vi "loadSTL.vi"(10 "STLname":string, 11 "Job Directory":path) -> (2 "STLpath":path, 3 "SceneObject out":refnum<vi>)   [LabVIEW 2022 SP3]
uses:
  <vilib>/Utility/miscctls.llb/LVRGBAColorTypeDef.ctl
  <vilib>/picture/3D Picture Control/Object/Create Object (name).vi
  <vilib>/picture/3D Picture Control/Object/Add Object (no reference).vi
  <vilib>/picture/3D Picture Control/NI_3D Picture Control.lvlib
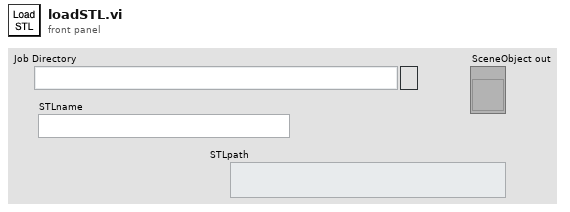
[diagram p1: front panel]
types:
  T1 = typedef "LVRGBAColorTypeDef.ctl" = cluster{"Red":sgl, "Green":sgl, "Blue":sgl, "Alpha":sgl}
  T2 = enum16{"Inherit Value", "Points", "Wireframe", "Polygons"}
  T3 = typedef "Triangle.ctl" = cluster{"V0":sgl[], "V1":sgl[], "V2":sgl[], "E0":sgl[], "E1":sgl[], "E2":sgl[], "n^":sgl[], "nE0^":sgl[], "nE1^":sgl[], "nE2^":sgl[]}
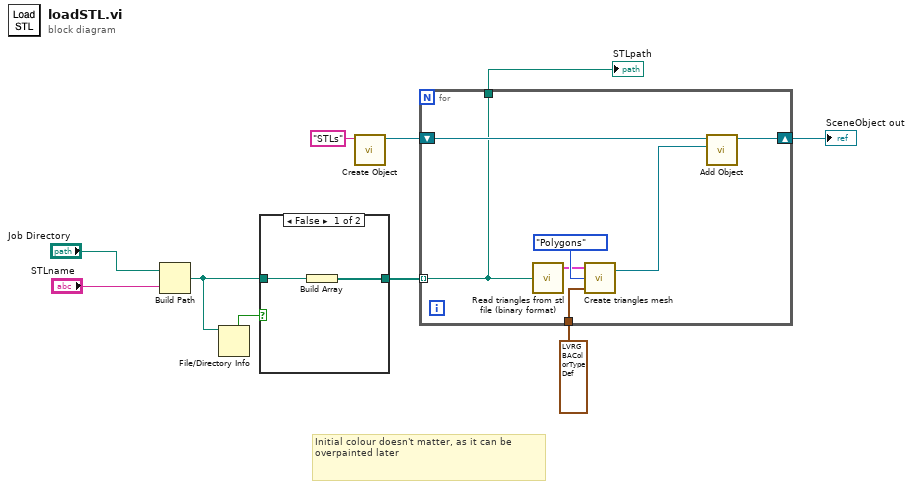
[diagram p0: block diagram]
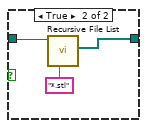
[diagram p2: hidden frame]
diagram:
  # "Initial colour doesn't matter, as it can be overpainted later"
  n1 = Build Path(base path="Job Directory", name or relative path="STLname") -> (appended path=w5:path)
  n2 = File/Directory Info(path=w5) -> (directory=w7:bool)  [unwired: 1 in, 6 out]
  n3 = case shown="False" w7 {
    tunnel: [w11 w14] -> w6
    tunnel: w5 -> [w12 w15]
    frame False {
      n4 = Build Array(w12) -> (w11:path[])
    }
    frame True {
      n5 = call <vilib>:"Recursive File List.vi"("pattern"="*.stl", "Folder Path"=w15) -> ("All Files in Dir"=w14:path[])  [unwired: 5 in, 4 out]
    }
  }
  n6 = call-poly <vilib>:"Create Object.vi"("Name"="STLs") -> ("Scene:New Object"=w8:refnum<vi>)  [unwired: 9 in, 1 out]
  n7 = for {
    tunnel: w6 -> [w17] mode=indexing
    shift-right: [w18] -> w1
    shift-left: w8 -> [w19]
    tunnel: [w17] -> w4
    tunnel: T1 {"Red"=0.7, "Green"=0.7, "Blue"=0.7, "Alpha"=1.0} ("Colour") -> [w16]
    n8 = call "Read triangles from stl file (binary format).vi"("STL file path"=w17) -> ("Triangles array"=w21:T3[])  [unwired: 2 out]
    n9 = call "Create triangles mesh.vi"("Colour"=w16, "Render mode"=T2."Polygons", "Triangles array"=w21) -> ("Triangle mesh out"=w20:refnum<vi>)  [unwired: 1 out]
    n10 = call-poly <vilib>:"Add Object.vi"("New Object In"=w20, "Scene Object In"=w19) -> ("Scene Object Out"=w18:refnum<vi>)  [unwired: 8 in, 1 out]
  }
  "SceneObject out" <- w1
  "STLpath" <- w4
